vi "Calc - PBADab.vi"(11 "00-00-9220":dbl[](array[numeric])) -> (1 "PBCOR":dbl, 2 "PBMeasP":dbl, 3 "PBADab":dbl)   [LabVIEW 2018, in "Controller (Host).lvlib"]
uses:
  Controller (Host).lvlib
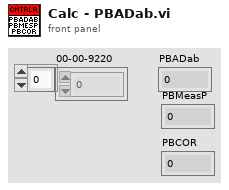
[diagram p1: front panel]
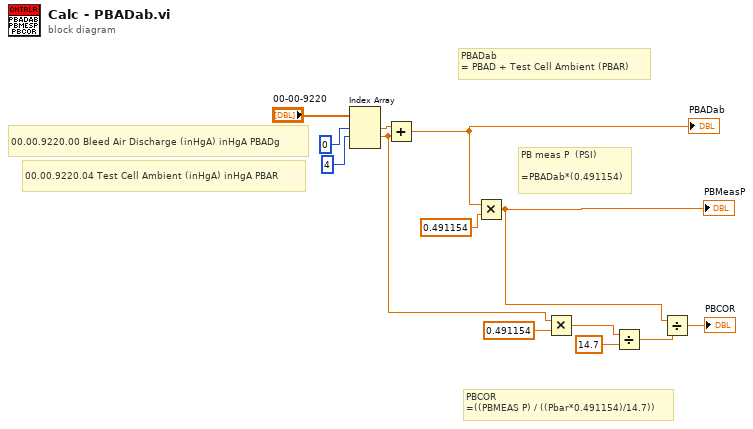
[diagram p0: block diagram]
diagram:
  # "PBCOR\n=((PBMEAS P) / ((Pbar*0.491154)/14.7))"
  # "PB meas P  (PSI)\n\n=PBADab*(0.491154)"
  # "00.00.9220.04\tTest Cell Ambient (inHgA)\tinHgA\tPBAR"
  # "PBADab \n= PBAD + Test Cell Ambient (PBAR)"
  # "00.00.9220.00\tBleed Air Discharge (inHgA)\tinHgA\tPBADg"
  n1 = Index Array(array="00-00-9220", index #1=0 ("index"), index #2=4 ("index")) -> (element #1=w13:dbl, element #2=w2:dbl)  [unwired: 1 in, 1 out]
  n2 = Add(x=w13, y=w2) -> (x+y=w8:dbl)
  "PBADab" <- w8
  n3 = Multiply(x=w8, y=0.491154) -> (x*y=w3:dbl)
  "PBMeasP" <- w3
  n4 = Multiply(x=w2, y=0.491154) -> (x*y=w4:dbl)
  n5 = Divide(x=w4, y=14.7) -> (x/y=w6:dbl)
  n6 = Divide(x=w3, y=w6) -> (x/y=→"PBCOR":dbl)
